vi "temp_test_vi.vi"() -> ()   [LabVIEW 2010, in "TrajectoryMH100122AODRAPS.lvclass"]
uses:
  TrajectoryMH100122AODRAPS.lvclass
  roi_visualization_cluster.ctl
panel:
  in  "roi in":T1(array[cluster])
  out "roi table out":T2[](array[typedef]) {"type" items=["point", "line", "poly line", "free line"]}
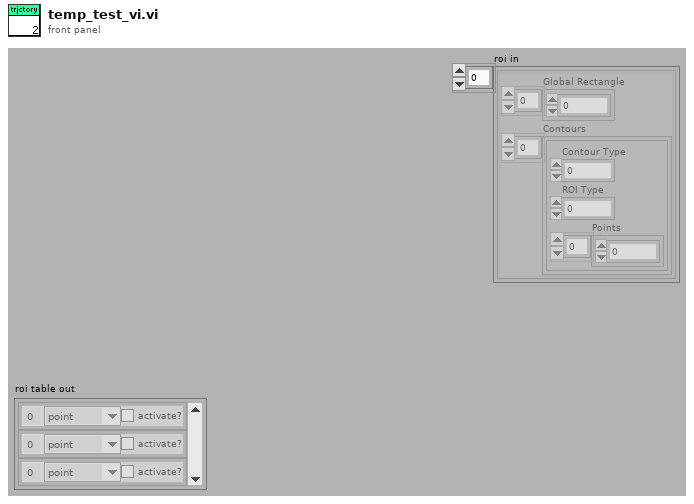
[diagram p1: front panel]
types:
  T1 = cluster{"Global Rectangle":i32[], "Contours":cluster{"Contour Type":u32, "ROI Type":u32, "Points":i32[]}[]}[]
  T2 = typedef "TrajectoryMH100122AODRAPS.lvclass/roi_visualization_cluster.ctl" = cluster{"counter":i32, "type":u16, "activation":bool}
  T3 = cluster{"Contour Type":u32, "ROI Type":u32, "Points":i32[]}[]
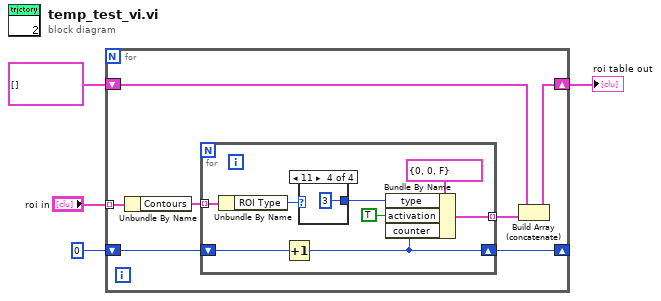
[diagram p0: block diagram]
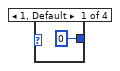
[diagram p2: hidden frame]
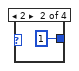
[diagram p3: hidden frame]
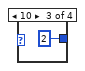
[diagram p4: hidden frame]
diagram:
  n1 = for {
    tunnel: "roi in" -> [w9] mode=indexing
    shift-right: [w10] -> _
    shift-left: 0 -> [w11]
    shift-right: [w7] -> w1
    shift-left: T2[] [] -> [w5]
    n2 = Unbundle By Name(w9) -> ("Contours"=w8:T3)
    n3 = for {
      tunnel: w8 -> [w17] mode=indexing
      shift-right: [w12] -> w10
      shift-left: w11 -> [w18]
      tunnel: [w14] -> w6 mode=indexing
      n4 = Unbundle By Name(w17) -> ("ROI Type"=w16:u32)
      n5 = Increment(x=w18) -> (x+1=w12:i32)
      n6 = case shown="11" w16 {
        tunnel: [u16 0 u16 1 u16 2 u16 3] -> w15
        frame 1, Default {
        }
        frame 2 {
        }
        frame 10 {
        }
        frame 11 {
        }
      }
      n7 = Bundle By Name(cluster=T2 {"counter"=0, "type"=0, "activation"=FALSE} ("System Cluster"), "type"=w15, "activation"=TRUE, "counter"=w12) -> (w14:T2)
    }
    n8 = Build Array (concatenate)(w5, w6) -> (w7:T2[])
  }
  "roi table out" <- w1
